vi "L_Run.vi"(8 "错误输入（无错误）":errorcluster, 11 "队列输入":refnum<queue>) -> ()   [LabVIEW 2018]
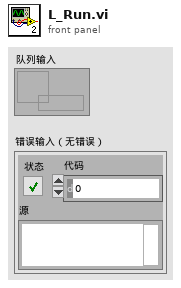
[diagram p1: front panel]
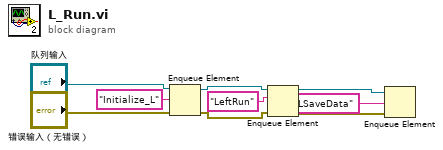
[diagram p0: block diagram]
diagram:
  n1 = Enqueue Element(queue="队列输入", element="Initialize_L", error in (no error)="错误输入（无错误）") -> (queue out=w1:refnum<queue>, error out=w2:errorcluster)  [unwired: 1 in, 1 out]
  n2 = Enqueue Element(queue=w1, element="LeftRun", error in (no error)=w2) -> (queue out=w5:refnum<queue>, error out=w4:errorcluster)  [unwired: 1 in, 1 out]
  n3 = Enqueue Element(queue=w5, element="LSaveData", error in (no error)=w4) -> ()  [unwired: 1 in, 3 out]
